vi "FIRSTSUBVIOUP.vi"() -> ()   [LabVIEW 2019]
panel:
  out "(A+B)/2":dbl
  in  "Numeric 2":dbl
  in  "Numeric":dbl
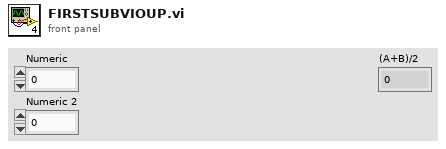
[diagram p1: front panel]
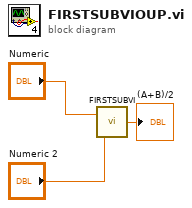
[diagram p0: block diagram]
diagram:
  n1 = call "FIRSTSUBVI.vi"("Numeric 2"="Numeric 2", "Numeric"="Numeric") -> ("(A+B)/2"=→"(A+B)/2":dbl)
